vi "Close.vi"(8 "error in (no error)":errorcluster, 11 "Client in":refnum<class "Client.lvclass">) -> (0 "error out":errorcluster, 3 "Client out":refnum<class "Client.lvclass">)   [LabVIEW 2020, in "Client.lvlib" / "Client.lvclass"]
uses:
  Client.lvclass
  Client.lvclass/Client.ctl
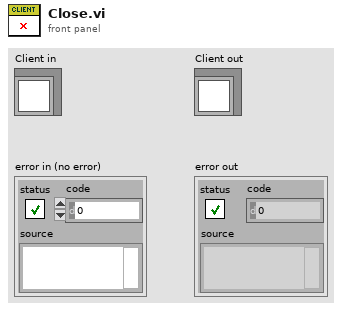
[diagram p1: front panel]
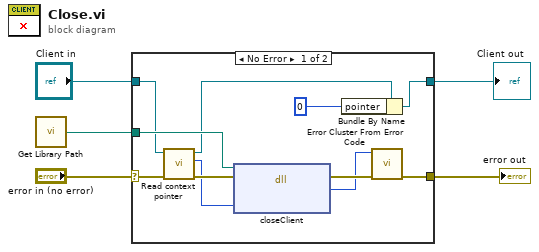
[diagram p0: block diagram]
diagram:
  n1 = call "Get Library Path.vi"() -> ("Path"=w1:path)  [unwired: 1 in]
  n2 = case shown="No Error" "error in (no error)" {
    selector: "error in (no error)" -> [w9 w17]
    tunnel: [w15 w17] -> w4
    tunnel: "Client in" -> [w8 w18]
    tunnel: [w13 w18] -> w2
    tunnel: w1 -> [w11 _]
    frame No Error {
      n3 = call "Read context pointer.vi"("error in (no error)"=w9, "Client in"=w8) -> ("error out"=w10:errorcluster, "client pointer"=w7:i64, "Client out"=w6:refnum<class "Client.lvclass">)  [unwired: 7 in]
      n4 = dll-call lib="?" fn="closeClient"(path in=w11, error in=w10, "client"=w7) -> (error out=w16:errorcluster, "ret_code"=w14:i32)  [unwired: 2 in, 1 out]
      n5 = Bundle By Name(cluster=w6, "pointer"=i64 0 ("context pointer")) -> (w13:refnum<class "Client.lvclass">)
      n6 = call <vilib>:"Error Cluster From Error Code.vi"("error in (no error)"=w16, "error code (0)"=w14) -> ("error out"=w15:errorcluster)  [unwired: 7 in]
    }
    frame Error {
    }
  }
  "error out" <- w4
  "Client out" <- w2
